vi "Initialize SPI Engine Resources 256-bit.vi"(8 "error in":errorcluster) -> (0 "error out":errorcluster, 3 "SPI Engine Resources 256-bit":T1={"To SPI Engine Data FIFO"="DLU To SPI Engine Data FIFO", "From SPI Engine Data FIFO"="SPI Engine to DLU Data FIFO", "Data to SPI Engine Cache Register"="Data to SPI Engine (Cache)", "SPI Transaction Settings Cache Register"="SPI PHY Settings to SPI Engine (Cache)"})   [LabVIEW 2015, in "SPI API.lvlib"]
doc: "This initializes FIFOs and Registers that are used by the SPI API for communication with the SPI Engine. This VI must be used to establish the references used by the other VIs in this API to send data to the SPI Engine."
uses:
  SPI API.lvlib
  Controls/SPI Engine Resources 256-bit.ctl
  <vilib>/rvi/DataTransferAndStorage/Container/Common/niFpgaContainerGetUniqueNameForEmu.vi
  <vilib>/rvi/DataTransferAndStorage/Container/Common/niFpgaContainerSetEmuInfo.vi
  <vilib>/rvi/eio/common/nirviEmuReportErrorAndStop.vi
  <vilib>/rvi/LocalResourceManager/LocalResourceManager.xnode
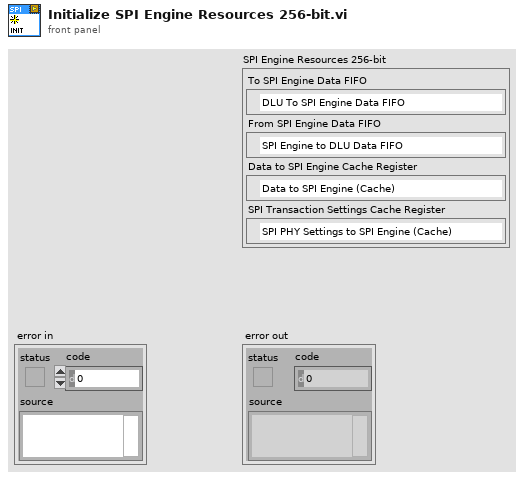
[diagram p1: front panel]
types:
  T1 = typedef "SPI API.lvlib/SPI Engine Resources 256-bit.ctl" = cluster{"To SPI Engine Data FIFO":refnum<k21>, "From SPI Engine Data FIFO":refnum<k21>, "Data to SPI Engine Cache Register":refnum<k21>, "SPI Transaction Settings Cache Register":refnum<k21>}
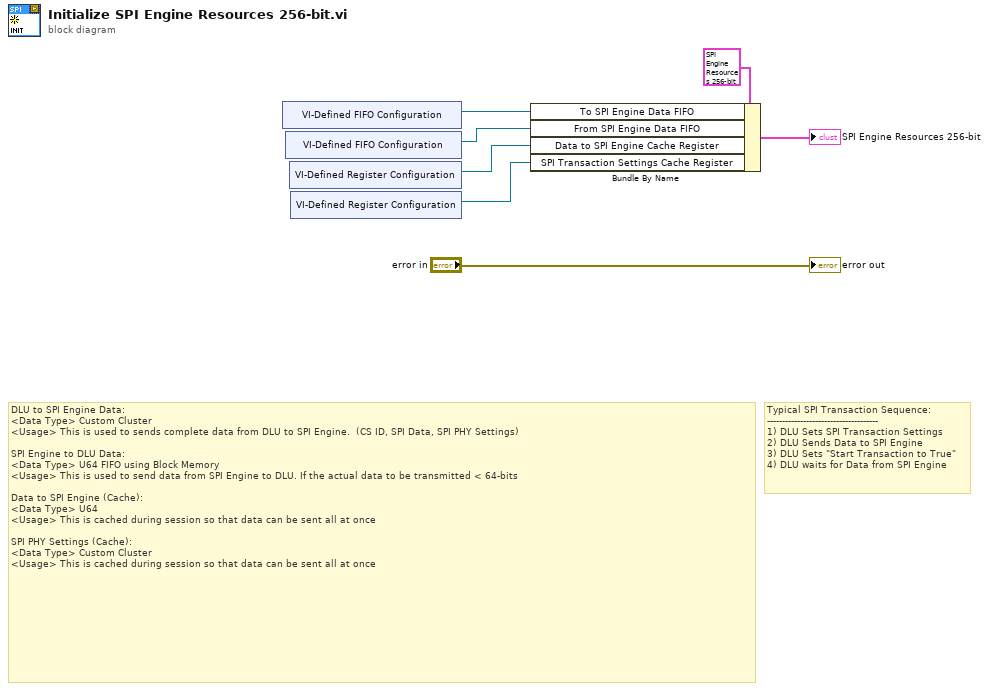
[diagram p0: block diagram]
diagram:
  # "Typical SPI Transaction Sequence:\n-------------------------------------\n1) DLU Sets SPI Transaction Settings\n2) DLU Sends Data to SPI Engine \n3) DLU Sets \"Start Transaction to True\"\n4) DLU waits for Data from SPI Engine"
  # "DLU to SPI Engine Data: \n<Data Type> Custom Cluster\n<Usage> This is used to sends complete data from DLU to SPI Engine.  (CS ID, SPI Data, SPI PHY Settings)\n\nSPI Engine to DLU Data: \n<Data Type> U64 FIFO using Block Memory\n<Usage> This is used to send data from SPI Engine to DLU. If the actual data to be transmitted < 64-bits\n\nData to SPI Engine (Cache):\n<Data Type> U64\n<Usage> This is cached during session so that data can be sent all at once\n\nSPI PHY Settings (Cache):\n<Data Type> Custom Cluster\n<Usage> This is cached during session so that data can be sent all at once"
  n1 = xnode "VI-Defined FIFO Configuration"() -> ("FIFO Out"=w4:refnum<k21>)
  n2 = xnode "VI-Defined FIFO Configuration"() -> ("FIFO Out"=w2:refnum<k21>)
  n3 = xnode ("VI-Defined Register Configuration")() -> ("Register Out"=w1:refnum<k21>)
  n4 = xnode ("VI-Defined Register Configuration")() -> ("Register Out"=w6:refnum<k21>)
  n5 = Bundle By Name(cluster=T1 {"To SPI Engine Data FIFO"="DLU To SPI Engine Data FIFO", "From SPI Engine Data FIFO"="SPI Engine to DLU Data FIFO", "Data to SPI Engine Cache Register"="Data to SPI Engine (Cache)", "SPI Transaction Settings Cache Register"="SPI PHY Settings to SPI Engine (Cache)"} ("Private Data"), "To SPI Engine Data FIFO"=w4, "From SPI Engine Data FIFO"=w2, "Data to SPI Engine Cache Register"=w1, "SPI Transaction Settings Cache Register"=w6) -> (→"SPI Engine Resources 256-bit":T1)
  "error out" <- "error in"
